vi "07-get-and_display_image.vi"() -> ()   [LabVIEW 2018, in "LV-0mq-Julia_roundtrip-lib.lvlib"]
uses:
  LV-0mq-Julia_roundtrip-lib.lvlib
  Server or client state.ctl
  Commands.ctl
  c965f866-6df0-488f-ad0f-a92a8fae8aa7.vi
  f9264f0d-2c2d-4a22-a0da-9e005a3dfb77.vi
  c965f866-6df0-488f-ad0f-a92a8fae8aa7.vi/9b4a1964-32a5-423d-9d7d-a559412da143.vi
  f9264f0d-2c2d-4a22-a0da-9e005a3dfb77.vi/17daa335-6bc4-4fc4-9d97-0b91b87d2130.vi
  c965f866-6df0-488f-ad0f-a92a8fae8aa7.vi/9b4a1964-32a5-423d-9d7d-a559412da143.vi/e3b3f1a0-ef46-4c90-961b-fe7e13c7819a.vi
  c965f866-6df0-488f-ad0f-a92a8fae8aa7.vi/9b4a1964-32a5-423d-9d7d-a559412da143.vi/78a69270-2d0f-484a-8c54-92d71671121a.vi
  c965f866-6df0-488f-ad0f-a92a8fae8aa7.vi/9b4a1964-32a5-423d-9d7d-a559412da143.vi/bbb7ffd9-f723-46a8-b782-2eb554ad1ab9.vi
  f9264f0d-2c2d-4a22-a0da-9e005a3dfb77.vi/17daa335-6bc4-4fc4-9d97-0b91b87d2130.vi/76ead16f-2b1e-4b12-ab0a-0cd1557670c1.vi
  f9264f0d-2c2d-4a22-a0da-9e005a3dfb77.vi/17daa335-6bc4-4fc4-9d97-0b91b87d2130.vi/3df4adb1-292d-40b8-aa92-f62b54c0127e.vi
  f9264f0d-2c2d-4a22-a0da-9e005a3dfb77.vi/17daa335-6bc4-4fc4-9d97-0b91b87d2130.vi/d48f62cf-a2ee-470f-a50d-38bd8fb0834d.vi
  check ID validity.vi
  bindata_descr to JSON.vi
  check cluster field names.vi
  concat JSON.vi
  build request.vi
  Parse server response.vi
  log jl exceptions.vi
  jl-scripts path.vi
panel:
  out "img_type":string
  out "picture":picture
  in  "select image":u16(ring) items=["autumn_leaves.png", "blobs.gif", "cameraman.tif", "chelsea.png", "coffee.png", "earth_apollo17.jpg", "fabio_color_256.png", "fabio_color_512.png", "fabio_gray_256.png", "fabio_gray_512.png", "hela-cells.tif", "house.tif", "jetplane.tif", "lake_color.tif", "lake_gray.tif", "lena_color_256.tif", "lena_color_512.tif", "lena_gray_256.tif", "lena_gray_512.tif", "lena_gray_16bit.png", "livingroom.tif", "lighthouse.png", "mandril_color.tif", "mandril_gray.tif", "mandrill.tiff", "m51.tif", "moonsurface.tiff", "mountainstream.png", "peppers_color.tif", "peppers_gray.tif", "pirate.tif", "resolution_test_512.tif", "resolution_test_1920.tif", "toucan.png", "walkbridge.tif", "woman_blonde.tif", "woman_darkhair.tif"]
  out "short error info":string
  in  "next":bool
  out "current error":errorcluster
  out "final error":errorcluster
  in  "stop":bool
  out "ZMQ timeout":bool
  out "Julia script file path":path
  out "temporary script path":path
  out "Jl Server state":T1
  # "If you don't see any received picture in this pane. check the scrollbars!"
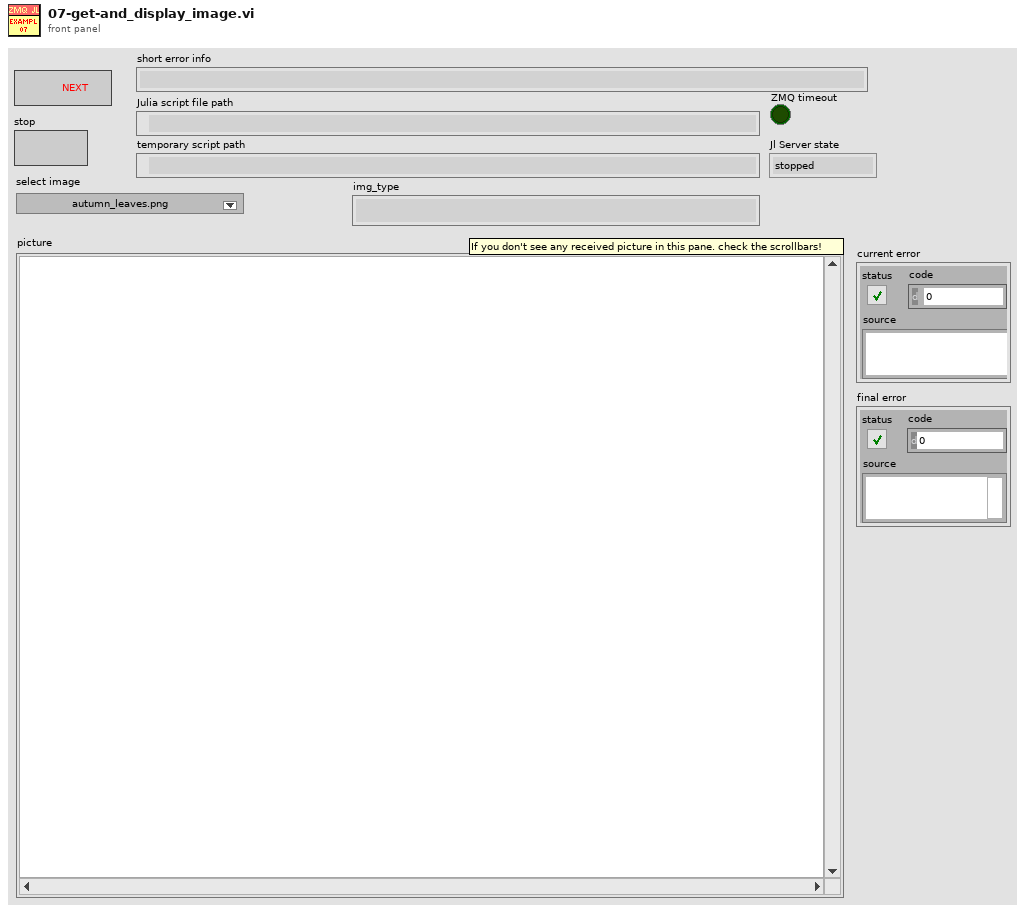
[diagram p1: front panel]
types:
  T1 = typedef "LV-0mq-Julia_roundtrip-lib.lvlib/Server or client state.ctl" = enum16{"stopped", "running", "unknown"}
  T2 = typedef "LV-0mq-Julia_roundtrip-lib.lvlib/Commands.ctl" = enum16{"Start Jl-server & Init LV-client", "Send request & Get response ", "Stop Jl-server & Cleanup LV-client", "Cleanup LV-client", "Start Jl-server", "Stop Jl-server", "Init LV-Client", "Cleanup LV-Client", "(not allowed)", "Set LV Client state", "Set Jl Server state", "set ZMQ timeout", "read ZMQ timeout", "read-out state"}
  T3 = typedef "LV-0mq-Julia_roundtrip-lib.lvlib/detailed error info.ctl" = cluster{"exception_or_info":string, "trace":T4[]}
  T4 = typedef "LV-0mq-Julia_roundtrip-lib.lvlib/StackFrame.ctl" = cluster{"frame_summary":string, "func":string, "linfo":string, "file":string, "line":i32, "pointer":u64, "from_c":bool, "inlined":bool}
  T5 = typedef "imagedata.ctl" = cluster{"image type":i32, "image depth":i32, "image":u8[], "mask":u8[], "colors":u32[], "Rectangle":cluster{"left":i16, "top":i16, "right":i16, "bottom":i16}}
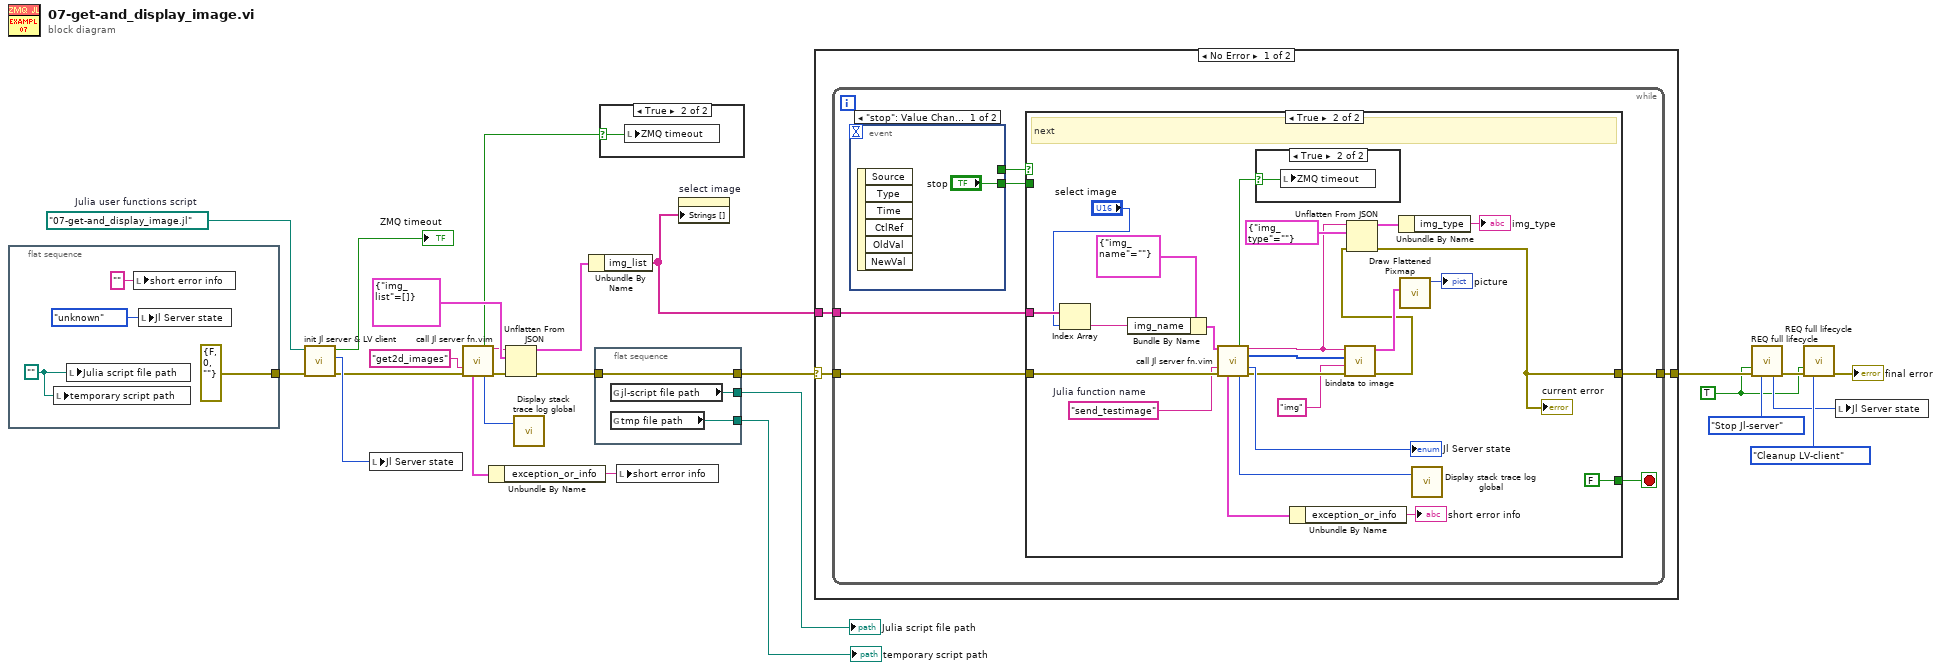
[diagram p0: block diagram]
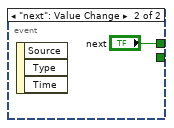
[diagram p3: hidden frame]
diagram:
  w5 = path "07-get-and_display_image.jl"  # Julia user functions script
  w17 = TRUE ("Force command")
  n1 = flat-sequence {
    tunnel: [errorcluster {"status"=FALSE, "code"=0, "source"=""} ("error in (no error)")] -> w2
    frame #0 {
      w28 = path ""
      n2 = local write "temporary script path"(w28) -> ()
      n3 = local write "Julia script file path"(w28) -> ()
      n4 = local write "short error info"("" ("short error info")) -> ()
      n5 = local write "Jl Server state"(Server_or_client_state."unknown" ("Jl Server state out")) -> ()
    }
  }
  n6 = call "init Jl server & LV client.vi"("error in (no error)"=w2, "Julia user functions script"=w5) -> ("error out"=w1:errorcluster, "Jl Server state out"=w3:T1, "timeout?"=→"ZMQ timeout":bool)  [unwired: 7 in]
  n7 = local write "Jl Server state"(w3) -> ()
  n8 = call "call Jl server fn.vim"("fun2call"="get2d_images", "error in (no error)"=w1) -> ("timeout?"=w10:bool, "JSON received"=w12:string, "detailed error info"=w9:T3, "return code"=w7:u8, "error out"=w11:errorcluster)  [unwired: 7 in, 2 out]
  n9 = Unbundle By Name(w9) -> ("exception_or_info"=w8:string)
  n10 = Unflatten From JSON(JSON string=w12, type and defaults=cluster{"img_list":string[]} {"img_list"=[]} ("parsed response"), error in (no error)=w11) -> (value=w14:cluster{"img_list":string[]}, error out=w16:errorcluster)  [unwired: 4 in]
  n11 = call "Display stack trace log global.vi"("return code"=w7) -> ()  [unwired: 3 in]
  n12 = Unbundle By Name(w14) -> ("img_list"=w6:string[])
  n13 = flat-sequence {
    tunnel: [w33] -> w21
    tunnel: w16 -> [w33]
    tunnel: [w32] -> w19
    tunnel: [w31] -> w20
    frame #0 {
      n14 = global read "jl-scripts path.vi" "jl-script file path"() -> (w32:path)
      n15 = global read "jl-scripts path.vi" "tmp file path"() -> (w31:path)
    }
  }
  n16 = case shown="True" w10 {
    selector: w10 -> [_ w34]
    frame False {
    }
    frame True {
      n17 = local write "ZMQ timeout"(w34) -> ()
    }
  }
  n18 = local write "short error info"(w8) -> ()
  n19 = property on="select image" class="Ring (strict)"("Strings []"=w6) -> ()  [unwired: 2 in, 2 out]
  n20 = case shown="No Error" w21 {
    selector: w21 -> [w36 w73]
    tunnel: [w37 w73] -> w26
    tunnel: w6 -> [w35 _]
    frame No Error {
      n21 = while {
        tunnel: w36 -> [w42]
        tunnel: [w43] -> w37
        tunnel: w35 -> [w38]
        stop <- w40 stop-if-true
        n22 = event shown="[0] \"stop\": Value Change" {
          selector: _ -> [_ _]
          dyn-events: _ -> [_ _]
          timeout: _ -> [_ _]
          tunnel: [_ "next"] -> w41
          tunnel: ["stop" _] -> w39
          event "stop": Value Change {
            n23 = event-data() -> ()  [unwired: 1 in, 6 out]
          }
          event "next": Value Change {
            n24 = event-data() -> ()  [unwired: 1 in, 3 out]
          }
        }
        n25 = case shown="True" w41 {
          tunnel: [w47 w49] -> w43
          tunnel: w42 -> [w47 w70]
          tunnel: [w46 FALSE ("stop this VI only")] -> w40
          tunnel: w39 -> [w46 _]
          tunnel: w38 -> [_ w61]
          frame False {
            # "stop"
          }
          frame True {
            w69 = "send_testimage"  # Julia function name
            # "next"
            n26 = Index Array(array=w61, index="select image") -> (element=w62:string)
            n27 = Bundle By Name(cluster=cluster{"img_name":string} {"img_name"=""} ("parsed response"), "img_name"=w62) -> (w59:cluster{"img_name":string})
            n28 = call "call Jl server fn.vim"("Arguments 1"=w59, "fun2call"=w69, "error in (no error)"=w70) -> ("timeout?"=w67:bool, "JSON received"=w48:string, "binary data received"=w55:u8[], "Jl Server state out"=→"Jl Server state":T1, "detailed error info"=w65:T3, "return code"=w66:u8, "error out"=w56:errorcluster)  [unwired: 6 in]
            n29 = case shown="True" w67 {
              selector: w67 -> [_ w72]
              frame False {
              }
              frame True {
                n30 = local write "ZMQ timeout"(w72) -> ()
              }
            }
            n31 = Unbundle By Name(w65) -> ("exception_or_info"=→"short error info":string)
            n32 = call "bindata to image.vi"("error in (no error)"=w56, "name"="img", "binary data in"=w55, "JSON in"=w48) -> ("error out"=w50:errorcluster, "img out"=w57:T5)  [unwired: 6 in]
            n33 = Unflatten From JSON(JSON string=w48, type and defaults=cluster{"img_type":string} {"img_type"=""}, error in (no error)=w50) -> (value=w52:cluster{"img_type":string}, error out=w49:errorcluster)  [unwired: 4 in]
            "current error" <- w49
            n34 = Unbundle By Name(w52) -> ("img_type"=→"img_type":string)
            n35 = call <vilib>:"Draw Flattened Pixmap.vi"("image data"=w57) -> ("new picture"=→"picture":picture)  [unwired: 8 in]
            n36 = call "Display stack trace log global.vi"("return code"=w66) -> ()  [unwired: 3 in]
          }
        }
      }
    }
    frame Error {
    }
  }
  n37 = call "REQ full lifecycle.vi"("Force command"=w17, "error in"=w26, "command"=Commands."Stop Jl-server") -> ("Jl Server state out"=w18:T1, "error out"=w24:errorcluster)  [unwired: 6 in, 5 out]
  n38 = call "REQ full lifecycle.vi"("Force command"=w17, "error in"=w24, "command"=Commands."Cleanup LV-client") -> ("error out"=→"final error":errorcluster)  [unwired: 6 in, 6 out]
  n39 = local write "Jl Server state"(w18) -> ()
  "temporary script path" <- w20
  "Julia script file path" <- w19
